vi "WireExistingErrorControl.vi"(7 "Control [t] / indicator [f]":bool, 8 "error in (no error)":errorcluster, 10 "Error terminals":T1, 11 "CaseStructure in":refnum<vi>) -> (0 "error out":errorcluster, 1 "Tunnel ref":refnum<vi>, 2 "Existing wiring used?":bool, 3 "CaseStructure (dup)":refnum<vi>)   [LabVIEW 2017, in "ErrorStructureDrawer.lvlib"]
doc: "If the error control/indicator was in the VI before the script started, check if it had a wire which now crosses into the new case structure (a tunnel). If so, return a boolean \"true\" and a reference to the tunnel.\n\nFor control only (not indicator), if a tunnel is found, use it as the selector terminal. If there are multiple tunnels, use the first one found."
uses:
  ErrorStructureDrawer.lvlib
  Controls/ErrorTerminals.ctl
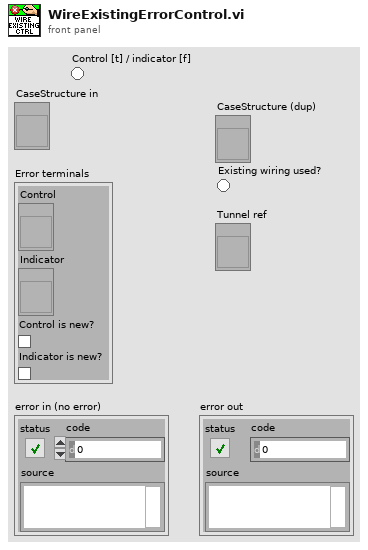
[diagram p1: front panel]
types:
  T1 = typedef "ErrorStructureDrawer.lvlib/ErrorTerminals.ctl" = cluster{"Control":refnum<vi>, "Indicator":refnum<vi>, "Control is new?":bool, "Indicator is new?":bool}
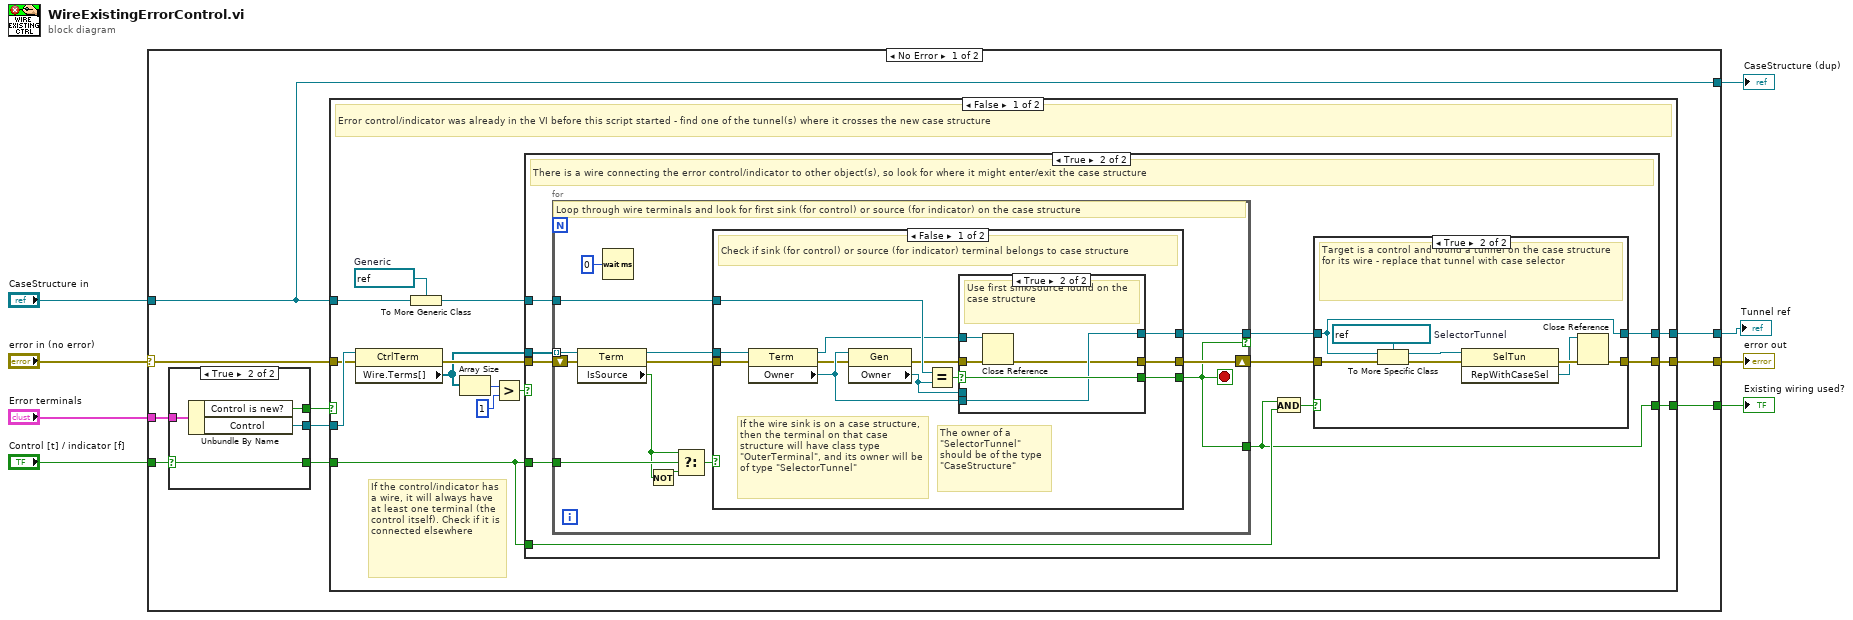
[diagram p0: block diagram]
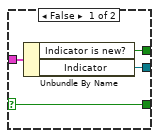
[diagram p2: hidden frame]
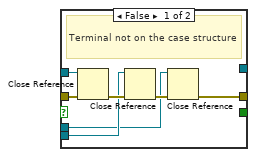
[diagram p5: hidden frame]
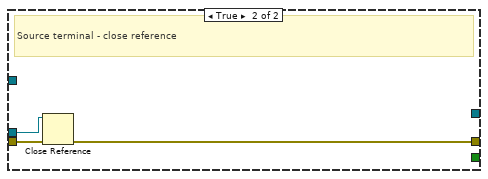
[diagram p6: hidden frame]
diagram:
  n1 = case shown="No Error" "error in (no error)" {
    selector: "error in (no error)" -> [w14 w105]
    tunnel: "CaseStructure in" -> [w13 w104]
    tunnel: [w18 w105] -> w7
    tunnel: "Error terminals" -> [w15 _]
    tunnel: [w13 w104] -> w4
    tunnel: [w12 _] -> w3
    tunnel: "Control [t] / indicator [f]" -> [w11 _]
    tunnel: [w9 _] -> w1
    frame No Error {
      n2 = case shown="True" w11 {
        selector: w11 -> [w19 w23]
        tunnel: [w20 w26] -> w17
        tunnel: [w21 w25] -> w16
        tunnel: w15 -> [w22 w24]
        tunnel: [w19 w23] -> w10
        frame False {
          n3 = Unbundle By Name(w22) -> ("Indicator is new?"=w21:bool, "Indicator"=w20:refnum<vi>)
        }
        frame True {
          n4 = Unbundle By Name(w24) -> ("Control is new?"=w25:bool, "Control"=w26:refnum<vi>)
        }
      }
      n5 = case shown="False" w16 {
        tunnel: w17 -> [w40 _]
        tunnel: w14 -> [w38 w103]
        tunnel: [w34 w103] -> w18
        tunnel: w13 -> [w35 _]
        tunnel: [w29 _] -> w12
        tunnel: w10 -> [w28 _]
        tunnel: [w27 _] -> w9
        frame False {
          w36 = refnum<vi> refnum  # Generic
          # "If the control/indicator has a wire, it will always have at least one terminal (the control itself). Check if it is connected elsewhere"
          # "Error control/indicator was already in the VI before this script started - find one of the tunnel(s) where it crosses the new case structure"
          n6 = property class="CtrlTerm"(reference=w40, error in=w38) -> (error out=w39:errorcluster, "Wire.Terms[]"=w31:refnum<vi>[])  [unwired: 1 out]
          n7 = To More Generic Class(target class=w36, reference=w35) -> (generic class reference=w37:refnum<vi>)
          n8 = Array Size(array=w31) -> (size(s)=w33:i32)
          n9 = Greater?(x=w33, y=1) -> (0:w30:bool)
          n10 = case shown="True" w30 {
            tunnel: w31 -> [_ w52]
            tunnel: w39 -> [w41 w51]
            tunnel: w37 -> [_ w50]
            tunnel: [w41 w47] -> w34
            tunnel: [_ w43] -> w29
            tunnel: w28 -> [_ w46]
            tunnel: w28 -> [_ w44]
            tunnel: [_ w42] -> w27
            frame False {
              # "There is no wire connecting the error control/indicator to other terminals, so do nothing"
            }
            frame True {
              # "There is a wire connecting the error control/indicator to other object(s), so look for where it might enter/exit the case structure"
              n11 = for {
                tunnel: w52 -> [w75] mode=indexing
                shift-right: [w72] -> w49
                shift-left: w51 -> [w71]
                tunnel: [w69] -> w48 if=w67
                tunnel: w50 -> [w68]
                tunnel: [w67] -> w43
                tunnel: w46 -> [w66]
                stop <- w67 stop-if-true
                # "Loop through wire terminals and look for first sink (for control) or source (for indicator) on the case structure"
                n12 = property class="Term"(reference=w75, error in=w71) -> (reference out=w73:refnum<vi>, error out=w74:errorcluster, "IsSource"=w64:bool)
                n13 = Wait (ms)(milliseconds to wait=u32 0) -> ()  [unwired: 1 out]
                n14 = Not(x=w64) -> (.not. x?=w63:bool)
                n15 = Select(t=w64, s=w66, f=w63) -> (s? t:f=w65:bool)
                n16 = case shown="False" w65 {
                  tunnel: w74 -> [w87 w102]
                  tunnel: w73 -> [w86 w101]
                  tunnel: [w81 _] -> w69
                  tunnel: [w82 w100] -> w72
                  tunnel: w68 -> [w85 _]
                  tunnel: [w80 _] -> w67
                  frame False {
                    # "The owner of a \"SelectorTunnel\" should be of the type \"CaseStructure\""
                    # "If the wire sink is on a case structure, then the terminal on that case structure will have class type \"OuterTerminal\", and its owner will be of type \"SelectorTunnel\""
                    # "Check if sink (for control) or source (for indicator) terminal belongs to case structure"
                    n17 = property class="Term"(reference=w86, error in=w87) -> (reference out=w83:refnum<vi>, error out=w78:errorcluster, "Owner"=w79:refnum<vi>)
                    n18 = property class="Gen"(reference=w79, error in=w78) -> (error out=w77:errorcluster, "Owner"=w76:refnum<vi>)  [unwired: 1 out]
                    n19 = Equal?(x=w85, y=w76) -> (x = y?=w84:bool)
                    n20 = case shown="True" w84 {
                      selector: w84 -> [_ w99]
                      tunnel: w77 -> [w94 w97]
                      tunnel: w83 -> [w93 w96]
                      tunnel: w79 -> [w91 w98]
                      tunnel: [w89 w95] -> w82
                      tunnel: [_ w99] -> w80
                      tunnel: [_ w98] -> w81
                      tunnel: w76 -> [w88 _]
                      frame False {
                        # "Terminal not on the case structure"
                        n21 = Close Reference(reference=w93, error in (no error)=w94) -> (error out=w92:errorcluster)
                        n22 = Close Reference(reference=w91, error in (no error)=w92) -> (error out=w90:errorcluster)
                        n23 = Close Reference(reference=w88, error in (no error)=w90) -> (error out=w89:errorcluster)
                      }
                      frame True {
                        # "Use first sink/source found on the case structure"
                        n24 = Close Reference(reference=w96, error in (no error)=w97) -> (error out=w95:errorcluster)
                      }
                    }
                  }
                  frame True {
                    # "Source terminal - close reference"
                    n25 = Close Reference(reference=w101, error in (no error)=w102) -> (error out=w100:errorcluster)
                  }
                }
              }
              n26 = And(x=w43, y=w44) -> (x .and. y?=w45:bool)
              n27 = case shown="True" w45 {
                tunnel: w49 -> [w54 w61]
                tunnel: w48 -> [w53 w55]
                tunnel: [w54 w56] -> w47
                tunnel: [w53 w55] -> w42
                frame False {
                  # "Indicator and/or no tunnel found, do nothing"
                }
                frame True {
                  w62 = refnum<vi> refnum  # SelectorTunnel
                  # "Target is a control and found a tunnel on the case structure for its wire - replace that tunnel with case selector"
                  n28 = To More Specific Class(target class=w62, reference=w55, error in=w61) -> (specific class reference=w60:refnum<vi>, error out=w59:errorcluster)
                  n29 = invoke class="SelTun" method="RepWithCaseSel"(reference=w60, error in=w59) -> (error out=w58:errorcluster, "RepWithCaseSel"=w57:refnum<vi>)  [unwired: 1 in, 1 out]
                  n30 = Close Reference(reference=w57, error in (no error)=w58) -> (error out=w56:errorcluster)
                }
              }
            }
          }
        }
        frame True {
          # "Error control/indicator is new - do nothing"
        }
      }
    }
    frame Error {
    }
  }
  "error out" <- w7
  "CaseStructure (dup)" <- w4
  "Existing wiring used?" <- w3
  "Tunnel ref" <- w1
